vi "CRYGenerate Pink Noise.vi"(6 "sampling info":cluster{"Fs":dbl, "#s":dbl}={"Fs"=51200.0, "#s"=1024.0} {"#s" format="%.2f"; "Fs" format="%.2p"}, 7 "reset signal (F)":bool, 8 "error in (no error)":errorcluster, 9 "seed":i32=-1, 11 "amplitude":dbl=1.0 format="%.2f") -> (0 "error out":errorcluster, 3 "pink noise signal":waveform(dbl))   [LabVIEW 2013]
uses:
  <vilib>/measure/NI_MABase.lvlib
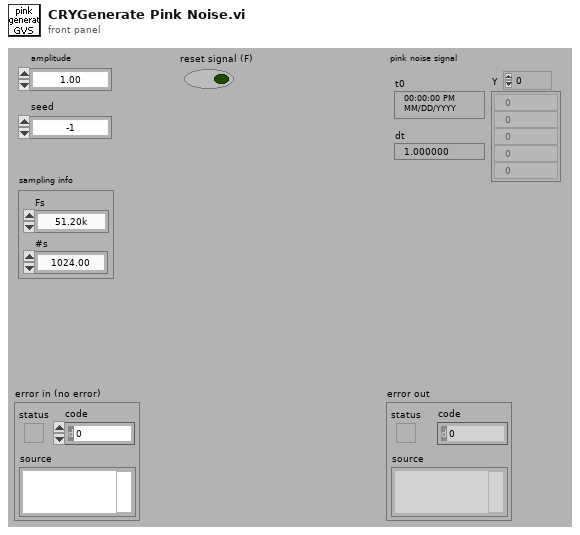
[diagram p1: front panel]
types:
  T1 = cluster{"lower cutoff freq":dbl, "higher cutoff freq":dbl, "order":i32}
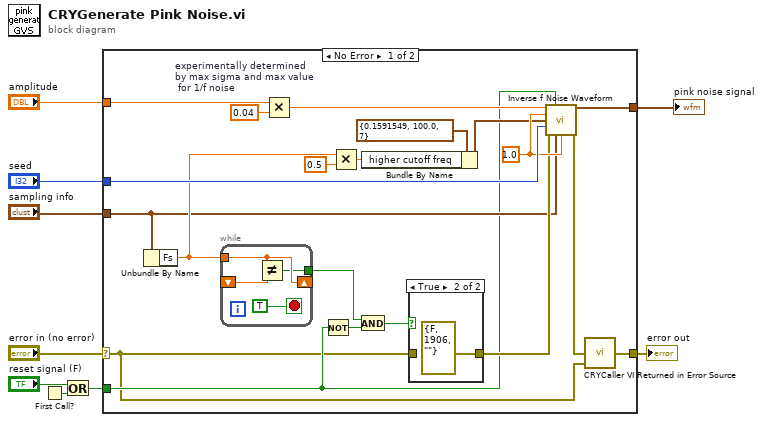
[diagram p0: block diagram]
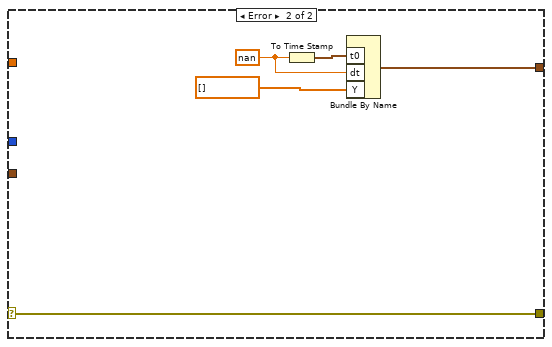
[diagram p3: hidden frame]
diagram:
  n1 = First Call?() -> (First Call?: T/F=w5:bool)
  n2 = Or(x="reset signal (F)", y=w5) -> (x .or. y?=w2:bool)
  n3 = case shown="No Error" "error in (no error)" {
    selector: "error in (no error)" -> [w11 w40]
    tunnel: [w10 w40] -> w8
    tunnel: "sampling info" -> [w17 _]
    tunnel: [w25 w39] -> w6
    tunnel: "amplitude" -> [w29 _]
    tunnel: "seed" -> [w27 _]
    tunnel: w2 -> [w14 _]
    frame No Error {
      w24 = 1.0 ("exponent")
      w28 = 0.04  # experimentally determined by max sigma and max value  for 1/f noise
      n4 = Unbundle By Name(w17) -> ("Fs"=w19:dbl)
      n5 = while {
        tunnel: [w30] -> w16
        tunnel: w19 -> [w32]
        shift-left: _ -> [w31]
        shift-right: [w32] -> _
        stop <- TRUE stop-if-true
        n6 = Not Equal?(x=w32, y=w31) -> (x != y?=w30:bool)
      }
      n7 = Multiply(x=w29, y=w28) -> (x*y=w26:dbl)
      n8 = Not(x=w14) -> (.not. x?=w13:bool)
      n9 = Multiply(x=w19, y=0.5) -> (x*y=w21:dbl)
      n10 = And(x=w16, y=w13) -> (x .and. y?=w15:bool)
      n11 = Bundle By Name(cluster=T1 {"lower cutoff freq"=0.1591549, "higher cutoff freq"=100.0, "order"=7} ("filter specifications"), "higher cutoff freq"=w21) -> (w20:T1)
      n12 = case shown="True" w15 {
        tunnel: w11 -> [w34 _]
        tunnel: [w34 errorcluster {"status"=FALSE, "code"=1906, "source"=""} ("error IO")] -> w18
        frame False {
        }
        frame True {
        }
      }
      n13 = call <vilib>:"Inverse f Noise Waveform.vi"("noise density"=w26, "reset signal (F)"=w14, "exponent"=w24, "filter specifications"=w20, "seed"=w27, "error in (no error)"=w18, "sampling info"=w17, "reference freq (Hz)"=w24) -> ("signal out"=w25:waveform(dbl), "error out"=w12:errorcluster)  [unwired: 6 out]
      n14 = call "CRYCaller VI Returned in Error Source.vi"("warning input to caller"=w11, "error in (no error)"=w12) -> ("error out"=w10:errorcluster)  [unwired: 3 out]
    }
    frame Error {
      w36 = nan ("t0")
      n15 = To Time Stamp(1:w36) -> (0:w37:timestamp)
      n16 = Bundle By Name("t0"=w37, "dt"=w36, "Y"=dbl[] []) -> (w39:waveform(dbl))  [unwired: 1 out]
    }
  }
  "error out" <- w8
  "pink noise signal" <- w6
